vi "AssertChannelLoopback.vi"(4 "Tolerance":dbl=0.01 format="%#_13g", 6 "Value":dbl, 7 "Delay Time (s)":dbl=0.1 format="%#_13g", 8 "error in (no error)":errorcluster, 9 "Read Channel":string, 10 "Write Channel":string, 11 "VeriStand Test Case in":refnum<class "VeriStandTestCase.lvclass">) -> (0 "error out":errorcluster, 3 "VeriStand Test Case out":refnum<class "VeriStandTestCase.lvclass">)   [LabVIEW 2015, in "VeriStandTestCase.lvclass"]
uses:
  VeriStandTestCase.lvclass
  VeriStandTestCase.lvclass/VeriStandTestCase.ctl
  <vilib>/NI Veristand/Execution/Workspace/NI VeriStand - Set Single Channel Value.vi
  <vilib>/NI Veristand/Execution/Workspace/NI VeriStand - Get Single Channel Value.vi
  <vilib>/NI VeriStand/Execution/Workspace/NI_VS Workspace ExecutionAPI.lvlib
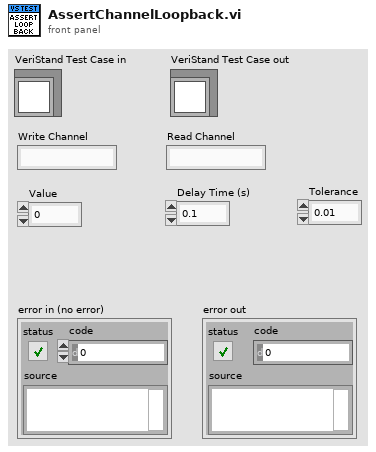
[diagram p1: front panel]
types:
  T1 = typedef "NI_VS Workspace ExecutionAPI.lvlib/WorkspaceAPI.ctl" = refnum<k24>
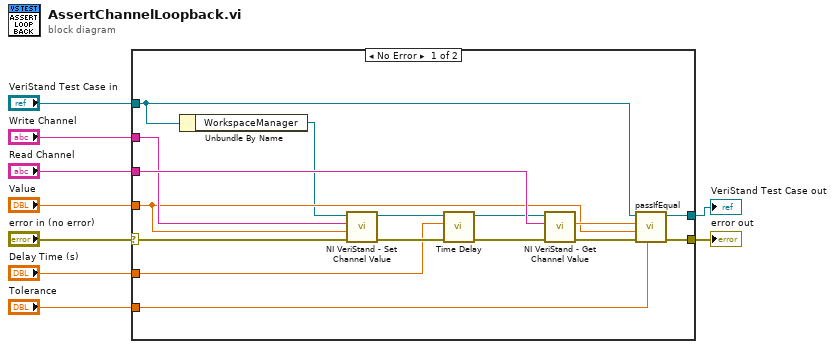
[diagram p0: block diagram]
diagram:
  n1 = case shown="No Error" "error in (no error)" {
    selector: "error in (no error)" -> [w18 w25]
    tunnel: [w24 w25] -> w9
    tunnel: "Read Channel" -> [w21 _]
    tunnel: "Write Channel" -> [w20 _]
    tunnel: "Value" -> [w19 _]
    tunnel: "Delay Time (s)" -> [w14 _]
    tunnel: "Tolerance" -> [w13 _]
    tunnel: "VeriStand Test Case in" -> [w11 w26]
    tunnel: [w12 w26] -> w1
    frame No Error {
      n2 = Unbundle By Name(w11) -> ("WorkspaceManager"=w10:T1)
      n3 = call-poly <vilib>:"NI VeriStand - Set Channel Value.vi"("error in (no error)"=w18, "Value"=w19, "Channel"=w20, "WorkspaceManager in"=w10) -> ("error out"=w16:errorcluster, "WorkspaceManager out"=w17:T1)  [unwired: 6 in]
      n4 = call "Time Delay"("error in (no error)"=w16, "Delay Time (s)"=w14) -> ("error out"=w15:errorcluster)  [unwired: 9 in]
      n5 = call-poly <vilib>:"NI VeriStand - Get Channel Value.vi"("error in (no error)"=w15, "Channel"=w21, "WorkspaceManager in"=w17) -> ("error out"=w23:errorcluster, "Value"=w22:dbl)  [unwired: 6 in, 1 out]
      n6 = call-dynamic "passIfEqual.vi"("delta (optional)"=w13, "error in (no error)"=w23, "y"=w19, "x"=w22, "TestCase in"=w11) -> ("error out"=w24:errorcluster, "TestCase out"=w12:refnum<class "VeriStandTestCase.lvclass">)  [unwired: 5 in]
    }
    frame Error {
    }
  }
  "error out" <- w9
  "VeriStand Test Case out" <- w1
